vi "Validate Supported Protocols.vi"(8 "error in (no error)":errorcluster, 11 "WebSocket In":refnum<class "WebSocket.lvclass">) -> (0 "error out":errorcluster, 3 "WebSocket out":refnum<class "WebSocket.lvclass">)   [LabVIEW 2021, in "WebSockets.lvlib" / "WebSocket.lvclass"]
doc: "Checks the headers for Sec-WebSocket-Protocol and if present, matches against the list of supported protocols specified by the server. If no protocols are supported, this VI will not return an error but the protocol will not returned.\nWebSockets 2.0.1.40\nSam Sharp - MediaMongrels Ltd\nCopyright (c) 2019, MediaMongrels Ltd"
uses:
  WebSocket.lvclass
  WebSocket.lvclass/WebSocket.ctl
  Read Protocols.vi
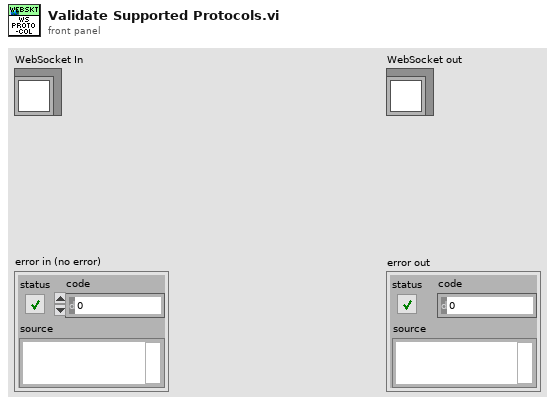
[diagram p1: front panel]
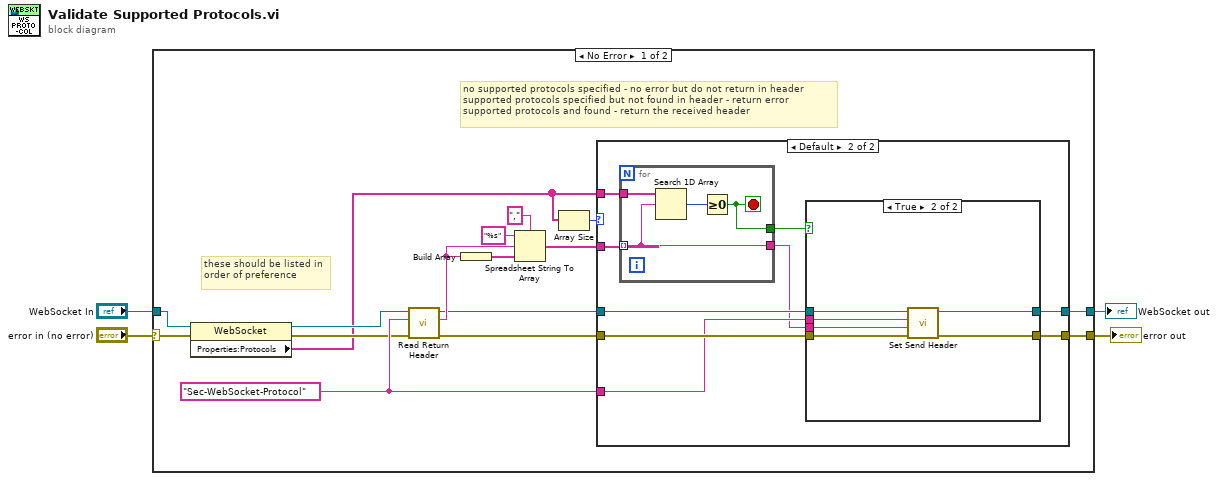
[diagram p0: block diagram]
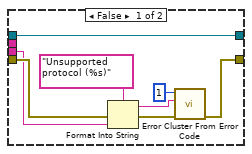
[diagram p3: hidden frame]
diagram:
  n1 = case shown="No Error" "error in (no error)" {
    selector: "error in (no error)" -> [w10 w51]
    tunnel: "WebSocket In" -> [w7 w50]
    tunnel: [w16 w50] -> w3
    tunnel: [w11 w51] -> w2
    frame No Error {
      w15 = "Sec-WebSocket-Protocol" ("Name")
      # "these should be listed in order of preference"
      # "no supported protocols specified - no error but do not return in header\nsupported protocols specified but not found in header - return error\nsupported protocols and found - return the received header"
      n2 = property class="WebSocket"(reference=w7, error in=w10) -> (reference out=w6:refnum<class "WebSocket.lvclass">, error out=w8:errorcluster, "Properties:Protocols"=w5:string[])
      n3 = call "Read Return Header.vi"("error in (no error)"=w8, "Name"=w15, "WebSocket in"=w6) -> ("error out"=w12:errorcluster, "Value"=w17:string, "WebSocket out"=w9:refnum<class "WebSocket.lvclass">)  [unwired: 5 in, 1 out]
      n4 = Build Array(w17) -> (w18:string[])
      n5 = Spreadsheet String To Array(delimiter (Tab)=",", format string="%s", spreadsheet string=w17, array type (2D Dbl)=w18) -> (array=w14:string[])
      n6 = Array Size(array=w5) -> (size(s)=w13:i32)
      n7 = case shown="Default" w13 {
        tunnel: w5 -> [_ w31]
        tunnel: w14 -> [_ w30]
        tunnel: [w21 w26] -> w16
        tunnel: w15 -> [_ w24]
        tunnel: w12 -> [w22 w29]
        tunnel: [w22 w27] -> w11
        tunnel: w9 -> [w21 w25]
        frame 0 {
          # "no supported protocols specified - allow any"
        }
        frame Default {
          n8 = for {
            tunnel: w30 -> [w48] mode=indexing
            tunnel: w31 -> [w49]
            tunnel: [w48] -> w23
            tunnel: [w46] -> w28
            stop <- w46 stop-if-true
            n9 = Search 1D Array(1D array=w49, element=w48) -> (index of element=w47:i32)  [unwired: 1 in]
            n10 = Greater Or Equal To 0?(x=w47) -> (x >= 0?=w46:bool)
          }
          n11 = case shown="True" w28 {
            tunnel: w29 -> [w33 w40]
            tunnel: [w35 w45] -> w27
            tunnel: [w34 w44] -> w26
            tunnel: w25 -> [w34 w43]
            tunnel: w24 -> [_ w42]
            tunnel: w23 -> [w32 w41]
            frame False {
              n12 = Format Into String(format string="Unsupported protocol (%s)", error in=w33, w32) -> (resulting string=w37:string, error out=w38:errorcluster)  [unwired: 1 in]
              n13 = call <vilib>:"Error Cluster From Error Code.vi"("error in (no error)"=w38, "error message (\"\")"=w37, "error code (0)"=1) -> ("error out"=w35:errorcluster)  [unwired: 6 in]
            }
            frame True {
              n14 = call "Set Send Header.vi"("error in (no error)"=w40, "Value"=w41, "Name"=w42, "WebSockets in"=w43) -> ("error out"=w45:errorcluster, "WebSockets out"=w44:refnum<class "WebSocket.lvclass">)  [unwired: 6 in]
            }
          }
        }
      }
    }
    frame Error {
    }
  }
  "WebSocket out" <- w3
  "error out" <- w2
